vi "DMMP_SetParameters.vi"(3 "Input Parameters":T1) -> (0 "Error?":bool, 1 "DMMP.lvclass":refnum<class "DMMP.lvclass">)   [LabVIEW 2014, in "DMMP.lvclass"]
uses:
  DMMP.lvclass
  DMMP.lvclass/DMMP.ctl
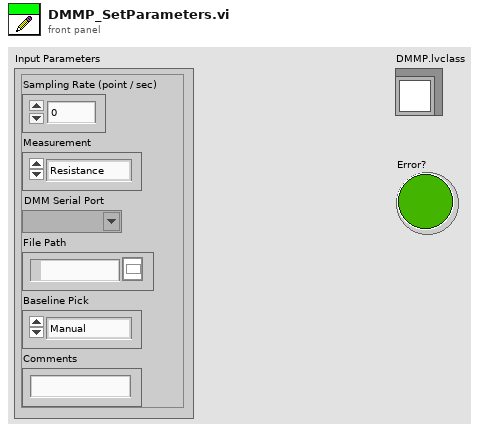
[diagram p1: front panel]
types:
  T1 = cluster{"Sampling Rate (point / sec)":u32, "Measurement":enum16{"Resistance", "Current"}, "DMM Serial Port":refnum<visa-resource-name>, "File Path":path, "Baseline Pick":enum16{"Manual", "Auto"}, "Comments":string}
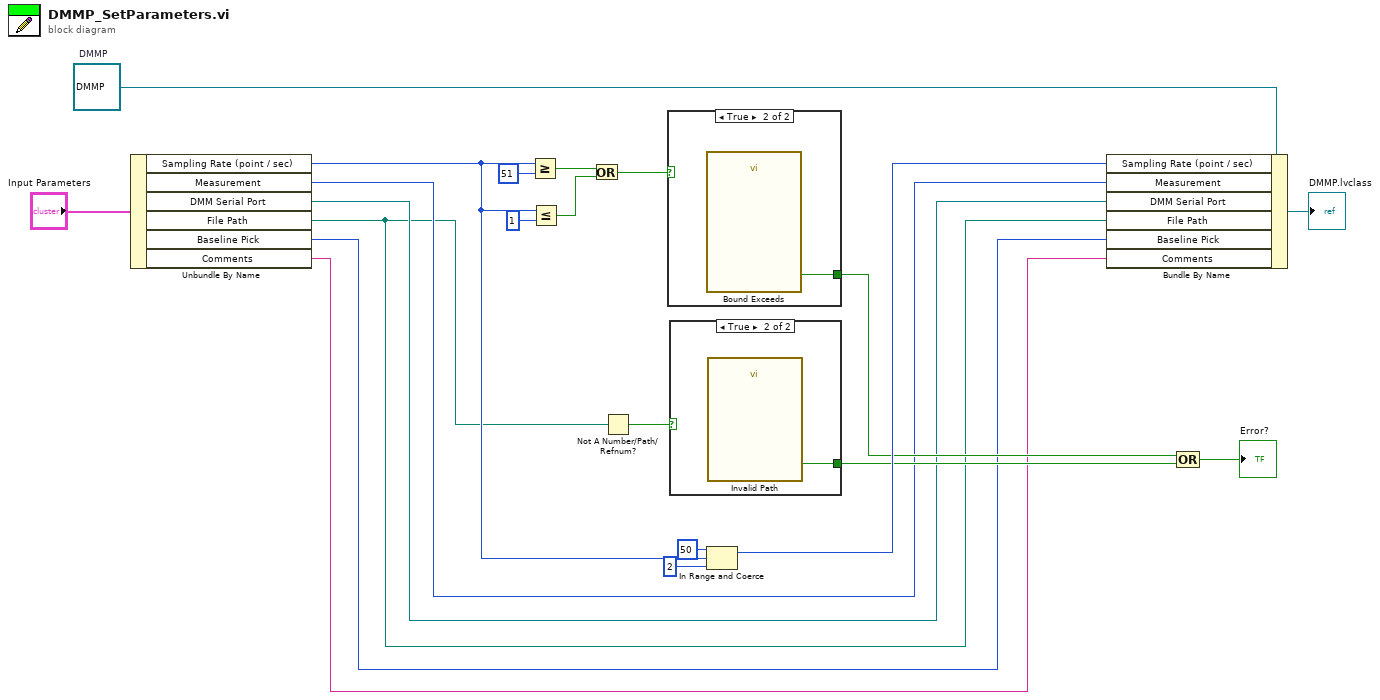
[diagram p0: block diagram]
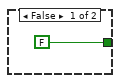
[diagram p2: hidden frame]
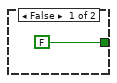
[diagram p3: hidden frame]
diagram:
  w21 = refnum<class "DMMP.lvclass"> refnum  # DMMP
  n1 = Unbundle By Name("Input Parameters") -> ("Sampling Rate (point / sec)"=w12:u32, "Measurement"=w6:enum16{"Resistance", "Current"}, "DMM Serial Port"=w5:refnum<visa-resource-name>, "File Path"=w4:path, "Baseline Pick"=w3:enum16{"Manual", "Auto"}, "Comments"=w2:string)
  n2 = Greater Or Equal?(x=w12, y=u32 51) -> (x >= y?=w16:bool)
  n3 = Less Or Equal?(x=w12, y=u32 1) -> (x <= y?=w15:bool)
  n4 = Or(x=w16, y=w15) -> (x .or. y?=w14:bool)
  n5 = Not A Number/Path/Refnum?(number/path/refnum=w4) -> (NaN/Path/Refnum?=w13:bool)
  n6 = case shown="True" w14 {
    tunnel: [FALSE ("OK") w23] -> w8
    frame False {
    }
    frame True {
      n7 = call "Bound Exceeds"() -> ("OK"=w23:bool)  [unwired: 10 in, 1 out]
    }
  }
  n8 = case shown="True" w13 {
    tunnel: [FALSE ("OK") w25] -> w7
    frame False {
    }
    frame True {
      n9 = call "Invalid Path"() -> ("OK"=w25:bool)  [unwired: 10 in, 1 out]
    }
  }
  n10 = In Range and Coerce(upper limit=u32 50, x=w12, lower limit=u32 2) -> (coerced(x)=w9:u32)  [unwired: 1 out]
  n11 = Bundle By Name(cluster=w21, "Sampling Rate (point / sec)"=w9, "Measurement"=w6, "DMM Serial Port"=w5, "File Path"=w4, "Baseline Pick"=w3, "Comments"=w2) -> (→"DMMP.lvclass":refnum<class "DMMP.lvclass">)
  n12 = Compound Arithmetic op=OR(w8, w7) -> (→"Error?":bool)
